vi "Write disconnected intervall.vi"(8 "error in (no error)":errorcluster, 10 "disconnected intervall":i32=1000, 11 "PolledDriver in":refnum<class "PolledDriver.lvclass">) -> (0 "error out":errorcluster, 3 "PolledDriver out":refnum<class "PolledDriver.lvclass">)   [LabVIEW 2013, in "PolledDriver.lvclass"]
doc: "Intervall (in milliseconds) between polls when the driver is NOT connected to the remote host"
uses:
  PolledDriver.lvclass
  PolledDriver.lvclass/PolledDriver.ctl
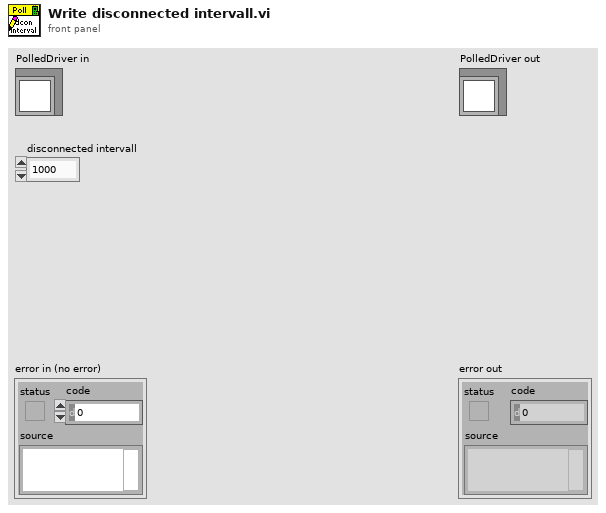
[diagram p1: front panel]
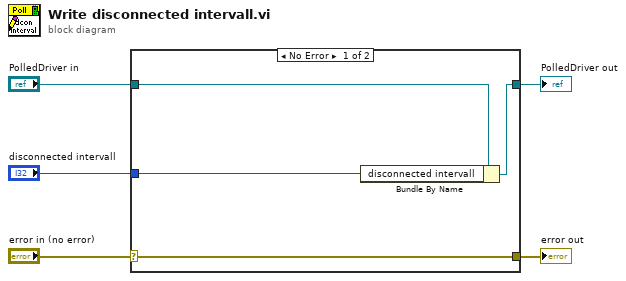
[diagram p0: block diagram]
diagram:
  n1 = case shown="No Error" "error in (no error)" {
    selector: "error in (no error)" -> [w9 w10]
    tunnel: [w9 w10] -> w4
    tunnel: [w7 w11] -> w2
    tunnel: "PolledDriver in" -> [w8 w11]
    tunnel: "disconnected intervall" -> [w6 _]
    frame No Error {
      n2 = Bundle By Name(cluster=w8, "disconnected intervall"=w6) -> (w7:refnum<class "PolledDriver.lvclass">)
    }
    frame Error {
    }
  }
  "error out" <- w4
  "PolledDriver out" <- w2
